vi "CRYASIO Close Cur Channel & Dev.vi"(8 "Limit":u32, 9 "isInput?":bool, 11 "Channel Out":u32 caption="Channel Index") -> ()   [LabVIEW 2013]
uses:
  CRYMisc vis settings global.vi
  Acquisition/SubVI/CRYAcquisition Global.vi
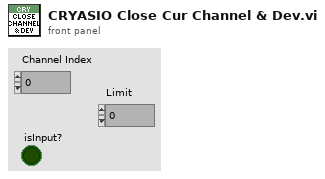
[diagram p1: front panel]
types:
  T1 = cluster{"Chn Name":string, "Count":i16, "Opend Idx":i16}[]
  T2 = cluster{"Chn Name":string, "Count":i16, "Opend Idx":i16}
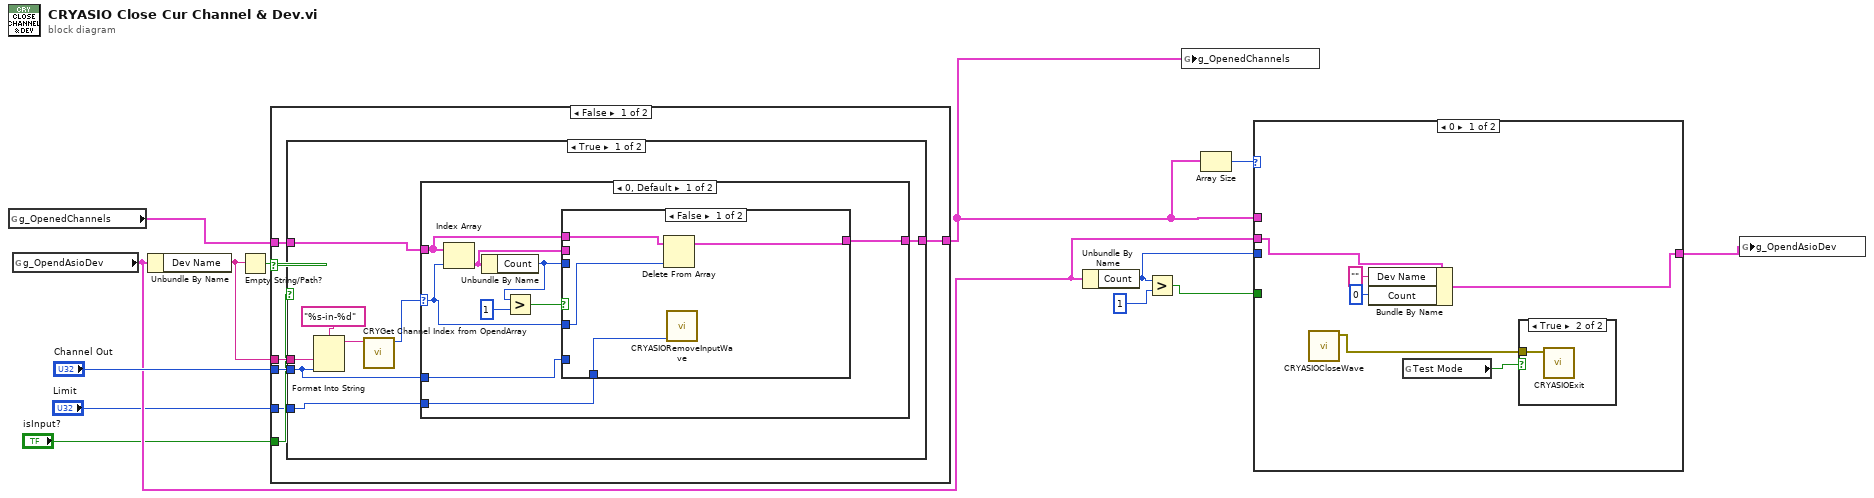
[diagram p0: block diagram]
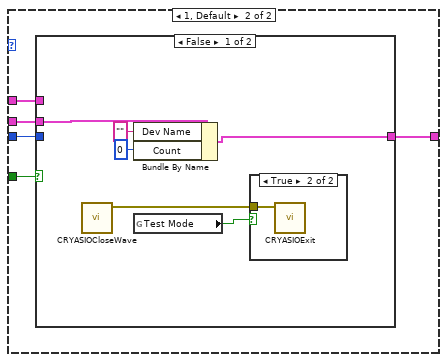
[diagram p3: hidden frame]
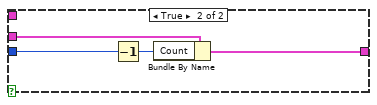
[diagram p5: hidden frame]
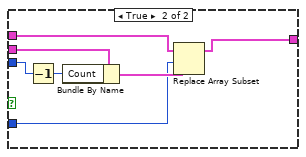
[diagram p6: hidden frame]
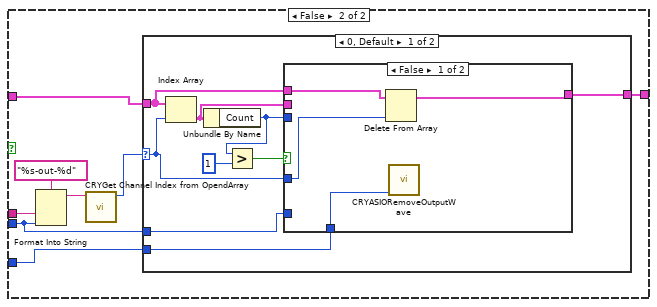
[diagram p8: hidden frame]
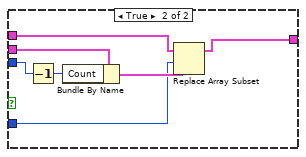
[diagram p9: hidden frame]
diagram:
  n1 = global read "CRYMisc vis settings global.vi" "g_OpenedChannels"() -> (w10:T1)
  n2 = global read "CRYMisc vis settings global.vi" "g_OpendAsioDev"() -> (w9:cluster{"Dev Name":string, "Count":i16})
  n3 = Unbundle By Name(w9) -> ("Dev Name"=w12:string)
  n4 = Empty String/Path?(string/path=w12) -> (empty?=w13:bool)
  n5 = case shown="False" w13 {
    tunnel: w12 -> [w19 _]
    tunnel: "Channel Out" -> [w17 _]
    tunnel: w10 -> [w18 w78]
    tunnel: [w16 w78] -> w2
    tunnel: "isInput?" -> [w15 _]
    tunnel: "Limit" -> [w14 _]
    frame False {
      n6 = case shown="True" w15 {
        tunnel: w19 -> [w26 w55]
        tunnel: w18 -> [w23 w52]
        tunnel: w17 -> [w22 w51]
        tunnel: [w21 w50] -> w16
        tunnel: w14 -> [w20 w49]
        frame True {
          n7 = Format Into String(format string="%s-in-%d", w26, w22) -> (resulting string=w25:string)  [unwired: 2 in, 1 out]
          n8 = call "CRYGet Channel Index from OpendArray.vi"("Channel Name"=w25) -> ("index of Channel"=w24:i32)  [unwired: 10 in]
          n9 = case shown="0, Default" w24 {
            selector: w24 -> [w31 _]
            tunnel: w23 -> [w32 w48]
            tunnel: [w30 w48] -> w21
            tunnel: w22 -> [w29 _]
            tunnel: w20 -> [w28 _]
            frame 0, Default {
              n10 = Index Array(array=w32, index=w31) -> (element=w33:T2)
              n11 = Unbundle By Name(w33) -> ("Count"=w34:i16)
              n12 = Greater?(x=w34, y=i16 1) -> (0:w35:bool)
              n13 = case shown="False" w35 {
                tunnel: w34 -> [_ w47]
                tunnel: w33 -> [_ w46]
                tunnel: w32 -> [w40 w44]
                tunnel: w31 -> [w39 w42]
                tunnel: [w38 w41] -> w30
                tunnel: w29 -> [_ _]
                tunnel: w28 -> [w37 _]
                frame False {
                  n14 = Delete From Array(array=w40, index=w39) -> (array with subset deleted=w38:T1)  [unwired: 1 in, 1 out]
                  n15 = call "CRYASIORemoveInputWave.vi"("OCI"=w37) -> ()  [unwired: 9 in, 2 out]
                }
                frame True {
                  n16 = Decrement(x=w47) -> (x-1=w45:i16)
                  n17 = Bundle By Name(cluster=w46, "Count"=w45) -> (w43:T2)
                  n18 = Replace Array Subset(array=w44, new element=w43, index=w42) -> (w41:T1)
                }
              }
            }
            frame -1 {
            }
          }
        }
        frame False {
          n19 = Format Into String(format string="%s-out-%d", w55, w51) -> (resulting string=w54:string)  [unwired: 2 in, 1 out]
          n20 = call "CRYGet Channel Index from OpendArray.vi"("Channel Name"=w54) -> ("index of Channel"=w53:i32)  [unwired: 10 in]
          n21 = case shown="0, Default" w53 {
            selector: w53 -> [w60 _]
            tunnel: w52 -> [w61 w77]
            tunnel: [w59 w77] -> w50
            tunnel: w51 -> [w58 _]
            tunnel: w49 -> [w57 _]
            frame 0, Default {
              n22 = Index Array(array=w61, index=w60) -> (element=w62:T2)
              n23 = Unbundle By Name(w62) -> ("Count"=w63:i16)
              n24 = Greater?(x=w63, y=i16 1) -> (0:w64:bool)
              n25 = case shown="False" w64 {
                tunnel: w63 -> [_ w76]
                tunnel: w62 -> [_ w75]
                tunnel: w61 -> [w69 w73]
                tunnel: w60 -> [w68 w71]
                tunnel: [w67 w70] -> w59
                tunnel: w58 -> [_ _]
                tunnel: w57 -> [w66 _]
                frame False {
                  n26 = Delete From Array(array=w69, index=w68) -> (array with subset deleted=w67:T1)  [unwired: 1 in, 1 out]
                  n27 = call "CRYASIORemoveOutputWave.vi"("OCI"=w66) -> ()  [unwired: 9 in, 2 out]
                }
                frame True {
                  n28 = Decrement(x=w76) -> (x-1=w74:i16)
                  n29 = Bundle By Name(cluster=w75, "Count"=w74) -> (w72:T2)
                  n30 = Replace Array Subset(array=w73, new element=w72, index=w71) -> (w70:T1)
                }
              }
            }
            frame -1 {
            }
          }
        }
      }
    }
    frame True {
    }
  }
  n31 = Unbundle By Name(w9) -> ("Count"=w5:i16)
  n32 = Greater?(x=w5, y=i16 1) -> (0:w6:bool)
  n33 = global write "CRYMisc vis settings global.vi" "g_OpenedChannels"(w2) -> ()
  n34 = Array Size(array=w2) -> (size(s)=w3:i32)
  n35 = case shown="0" w3 {
    tunnel: w9 -> [w82 w90]
    tunnel: [w81 w89] -> w8
    tunnel: w6 -> [_ w88]
    tunnel: w5 -> [_ w87]
    tunnel: w2 -> [_ w86]
    frame 0 {
      n36 = call "CRYASIOCloseWave.vi"() -> ("error out"=w79:errorcluster)  [unwired: 10 in, 1 out]
      n37 = Bundle By Name(cluster=w82, "Dev Name"="", "Count"=i16 0) -> (w81:cluster{"Dev Name":string, "Count":i16})
      n38 = global read "CRYAcquisition Global.vi" "Test Mode"() -> (w80:bool)
      n39 = case shown="True" w80 {
        tunnel: w79 -> [_ w85]
        frame False {
        }
        frame True {
          n40 = call "CRYASIOExit.vi"("error in (no error)"=w85) -> ()  [unwired: 9 in, 2 out]
        }
      }
    }
    frame 1, Default {
      n41 = case shown="False" w88 {
        tunnel: w87 -> [_ w101]
        tunnel: w90 -> [w96 w99]
        tunnel: [w93 w98] -> w89
        tunnel: w86 -> [_ _]
        frame False {
          n42 = call "CRYASIOCloseWave.vi"() -> ("error out"=w91:errorcluster)  [unwired: 10 in, 1 out]
          n43 = Bundle By Name(cluster=w96, "Dev Name"="", "Count"=i16 0) -> (w93:cluster{"Dev Name":string, "Count":i16})
          n44 = global read "CRYAcquisition Global.vi" "Test Mode"() -> (w92:bool)
          n45 = case shown="True" w92 {
            tunnel: w91 -> [_ w97]
            frame False {
            }
            frame True {
              n46 = call "CRYASIOExit.vi"("error in (no error)"=w97) -> ()  [unwired: 9 in, 2 out]
            }
          }
        }
        frame True {
          n47 = Decrement(x=w101) -> (x-1=w100:i16)
          n48 = Bundle By Name(cluster=w99, "Count"=w100) -> (w98:cluster{"Dev Name":string, "Count":i16})
        }
      }
    }
  }
  n49 = global write "CRYMisc vis settings global.vi" "g_OpendAsioDev"(w8) -> ()
